vi "rethinkdb_msg_error_str.vi"(8 "error in (no error)":errorcluster, 11 "message":string) -> (0 "error out":errorcluster, 3 "error":errorcluster)   [LabVIEW 2017]
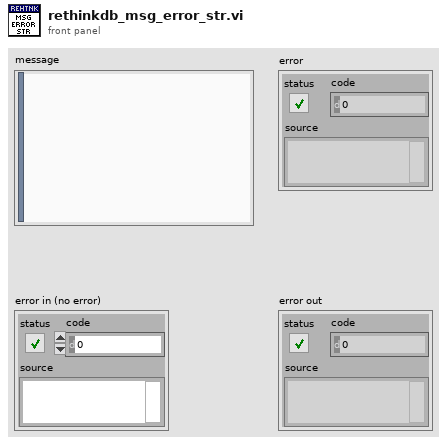
[diagram p1: front panel]
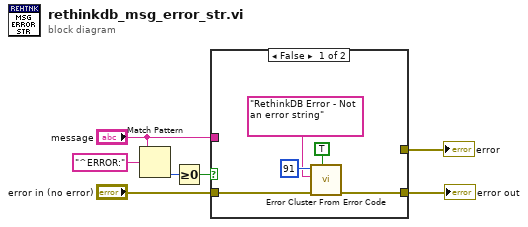
[diagram p0: block diagram]
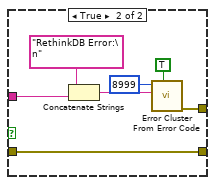
[diagram p2: hidden frame]
diagram:
  n1 = Match Pattern(string="message", regular expression="^ERROR:") -> (offset past match=w2:i32)  [unwired: 1 in, 3 out]
  n2 = Greater Or Equal To 0?(x=w2) -> (x >= 0?=w1:bool)
  n3 = case shown="False" w1 {
    tunnel: "error in (no error)" -> [w10 w19]
    tunnel: "message" -> [_ w18]
    tunnel: [w9 w19] -> w6
    tunnel: [_ w17] -> w4
    frame False {
      n4 = call <vilib>:"Error Cluster From Error Code.vi"("show call chain? (False)"=TRUE, "error in (no error)"=w10, "error message (\"\")"="RethinkDB Error - Not an error string" ("error message (\"\")"), "error code (0)"=91) -> ("error out"=w9:errorcluster)  [unwired: 5 in]
    }
    frame True {
      n5 = Concatenate Strings("RethinkDB Error:\n" ("error message (\"\")"), w18) -> (w13:string)
      n6 = call <vilib>:"Error Cluster From Error Code.vi"("show call chain? (False)"=TRUE, "error message (\"\")"=w13, "error code (0)"=8999) -> ("error out"=w17:errorcluster)  [unwired: 6 in]
    }
  }
  "error out" <- w6
  "error" <- w4
